vi "模态分析使用版2.vi"() -> ()   [LabVIEW 2014]
uses:
  <vilib>/Analysis/4window.llb/windowTd.ctl
  <vilib>/Utility/error.llb/DialogType.ctl
  <vilib>/DAQmx/read.llb/DAQmx Read (Analog 1D Wfm NChan NSamp).vi
  <vilib>/DAQmx/create/channels.llb/DAQmx Create Channel (AI-Voltage-Basic).vi
  <vilib>/DAQmx/configure/timing.llb/DAQmx Timing (Sample Clock).vi
  <vilib>/DAQmx/miscellaneous.llb/DAQmx Fill In Error Info.vi
  <vilib>/Waveform/WDTOps.llb/WDT Number of Waveform Samples DBL.vi
  <vilib>/Waveform/WDTOps.llb/WDT Append Waveforms DBL.vi
  <vilib>/Waveform/WDTOps.llb/WDT Get Waveform Subset DBL.vi
  <vilib>/Analysis/NI_AALPro.lvlib
panel:
  out "FRF magnifitude":cluster{"f0":dbl, "df":dbl, "magnitude":dbl[]}(graph)
  out "相关函数":cluster{"f0":dbl, "df":dbl, "magnitude":dbl[]}(graph)
  out "FRF Phase":cluster{"f0":dbl, "df":dbl, "magnitude":dbl[]}(graph)
  in  "DAQmx物理通道":tag
  in  "input terminal configuration 2":i32(ring)=-1 caption="输入接线端配置" items=["默认"=-1, "RSE"=10083, "NRSE"=10078, "差分"=10106, "伪差分"=12529]
  in  "DAQmx物理通道 2":tag
  in  "input terminal configuration 3":i32(ring)=-1 caption="输入接线端配置" items=["默认"=-1, "RSE"=10083, "NRSE"=10078, "差分"=10106, "伪差分"=12529]
  in  "rate 2":dbl=1000.0 caption="速率" format="%0.2f"
  in  "sample mode 2":i32(ring)=10178 caption="采样模式" items=["有限采样"=10178, "连续采样"=10123, "硬件定时单点"=12522]
  in  "number of samples per channel 2":i32=-1 caption="每通道采样数"
  in  "最小采集电压值 2":dbl=-10.0 format="%#_g  V"
  in  "最大采集电压值  2":dbl=10.0 format="%#_g  V"
  in  "units 2":i32(ring)=10348 caption="单位" items=["伏特"=10348, "来自自定义换算"=10065]
  in  "units 3":i32(ring)=10348 caption="单位" items=["伏特"=10348, "来自自定义换算"=10065]
  in  "averaging parameters":T1={"averaging mode"=enum."No averaging", "weighting mode"=enum."Exponential", "number of averages"=10} caption="平均参数" {"number of averages" min=1}
  in  "window":T2=1 caption="窗" items=["矩形"=0, "Hanning"=1, "Hamming"=2, "Blackman-Harris"=3, "Exact Blackman"=4, "Blackman"=5, "Flat Top"=6, "4阶Blackman-Harris "=7, "7阶Blackman-Harris"=8, "Low Sidelobe"=9, "Blackman Nuttall"=11, "三角"=30, "Bartlett-Hanning"=31, "Bohman"=32, "Parzen"=33, "Welch"=34, "Kaiser"=60, "Dolph-Chebyshev"=61, "高斯"=62]
  in  "view":T3 caption="查看"
  in  "FRF Mode":enum16{"H1", "H2", "H3"}(ring) caption="FRF模式"
  in  "删除上一次波形":bool
  out "激振信号":waveform(dbl)(graph)
  out "响应信号":waveform(dbl)(graph)
  out "激振信号 3":waveform(dbl)[](graph)
  in  "数值":i32
  out "激振信号 4":waveform(dbl)[](graph)
  in  "阈值":dbl=-1.0
  in  "预触发长度":i32=-1
  in  "激振通道":i32=-1
  in  "激振传感器灵敏度":dbl=-1.0
  in  "采集次数":i32=-1 caption="预触发长度"
  in  "停止按钮":bool
  in  "激振计数":i32=-1 caption="预触发长度"
  out "激振信号 2":waveform(dbl)[](graph)
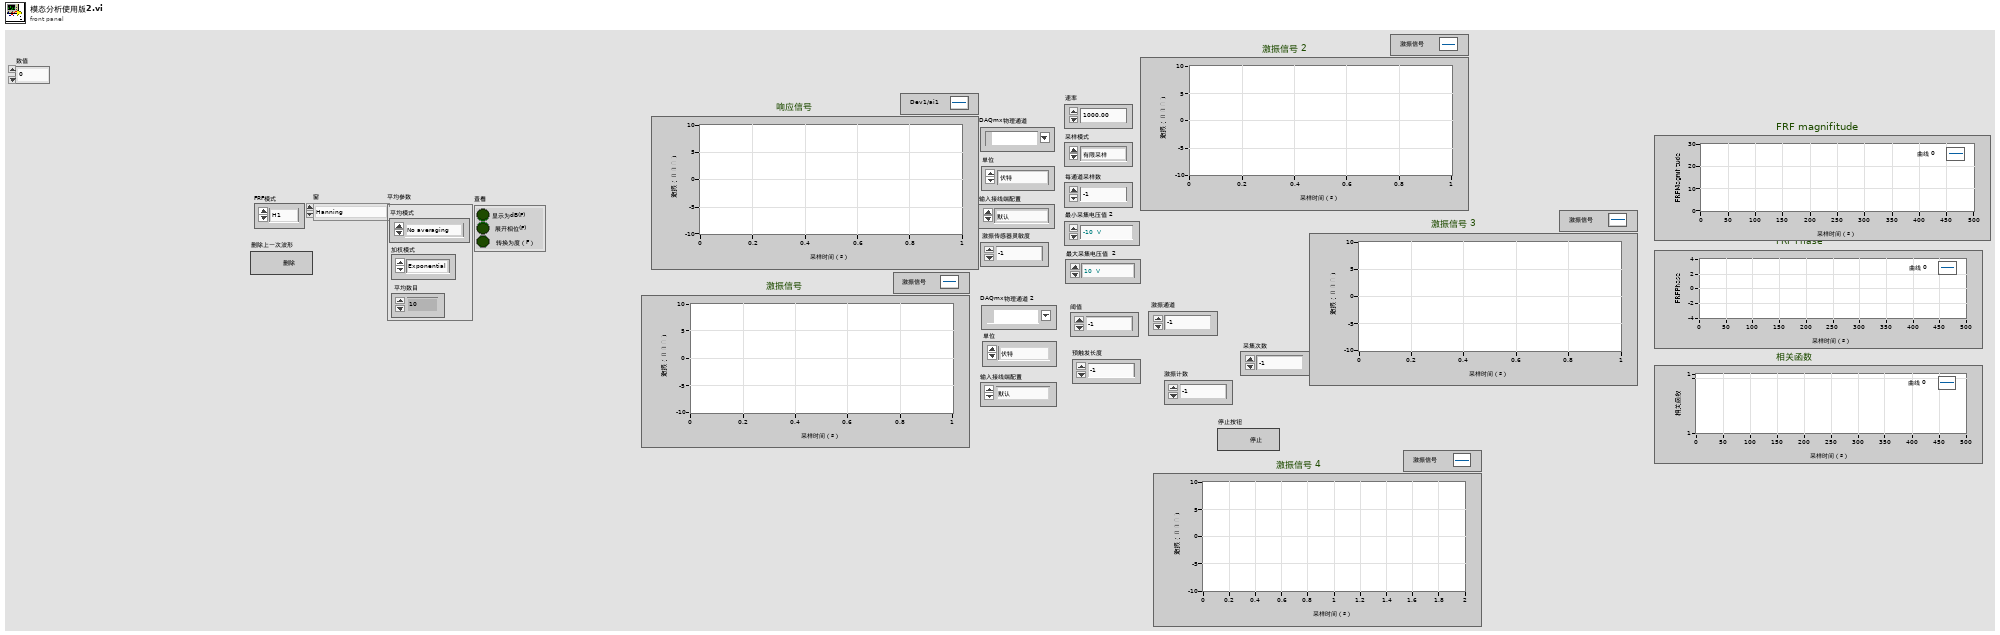
[diagram p1: front panel]
types:
  T1 = cluster{"averaging mode":enum16{"No averaging", "Vector averaging", "RMS averaging", "Peak hold"}, "weighting mode":enum16{"Linear", "Exponential"}, "number of averages":u32}
  T2 = typedef "NI_AALPro.lvlib/windowTd.ctl" = u32
  T3 = cluster{"dB On (F)":bool, "unwrap phase (F)":bool, "convert to degree (F)":bool}
  T4 = typedef "DialogType.ctl" = u16
  T5 = cluster{"magnitude":cluster{"f0":dbl, "df":dbl, "magnitude":dbl[]}, "phase":cluster{"f0":dbl, "df":dbl, "phase":dbl[]}, "coherence":cluster{"f0":dbl, "df":dbl, "coherence":dbl[]}}
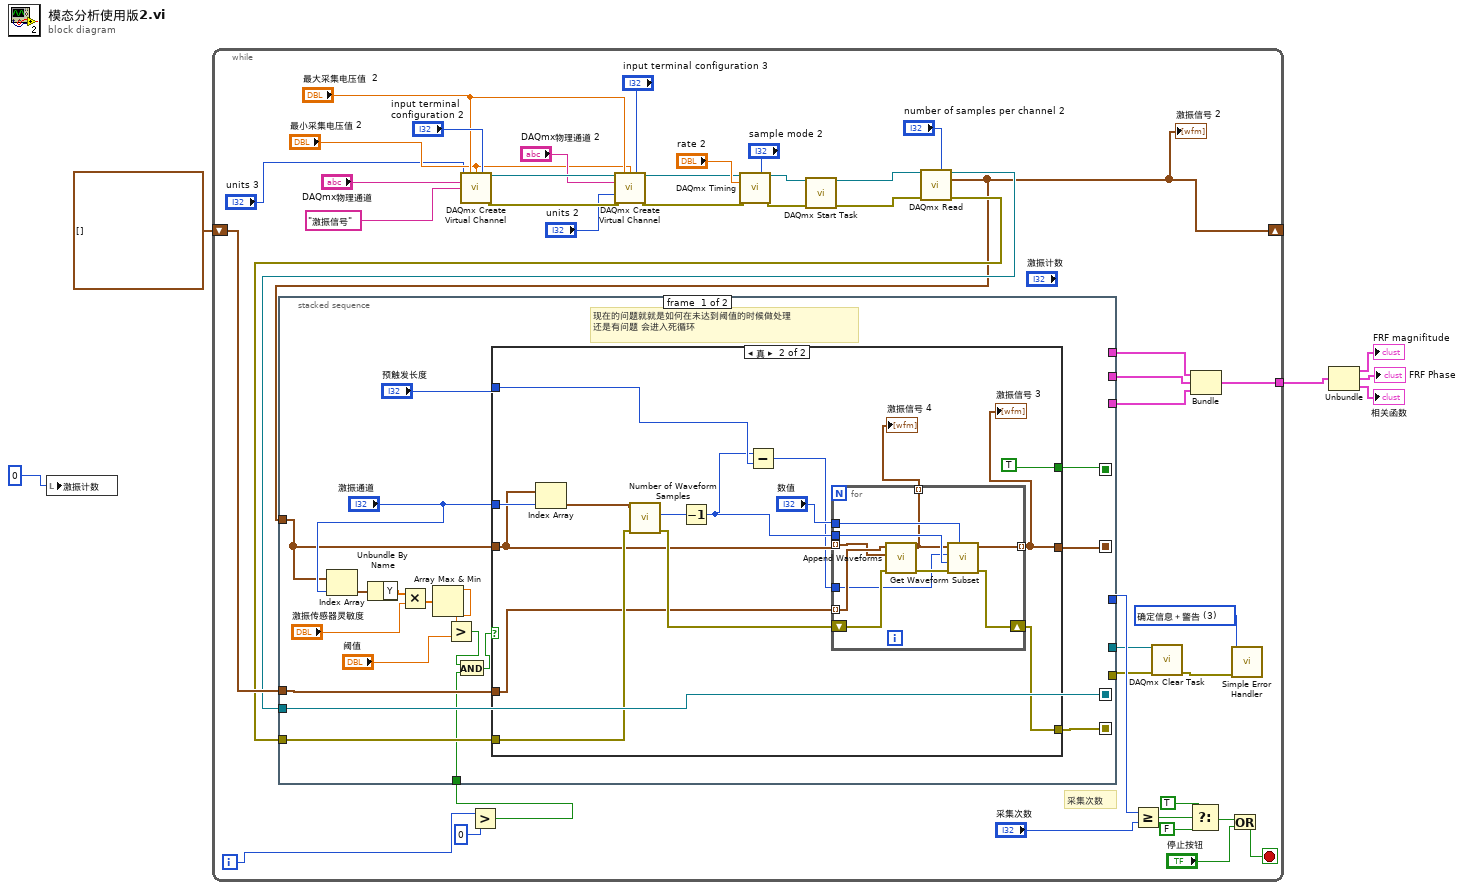
[diagram p0: block diagram]
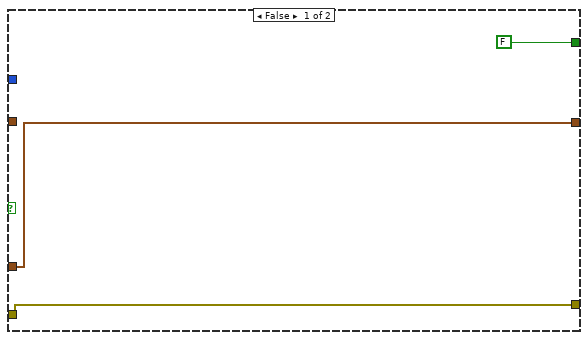
[diagram p2: hidden frame]
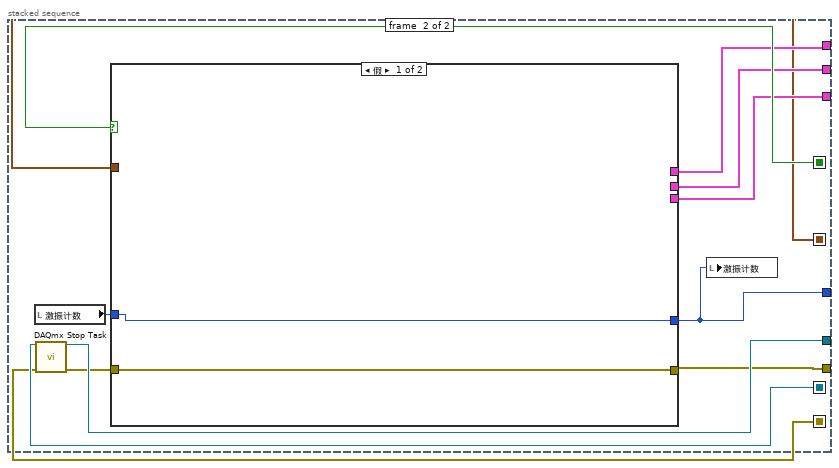
[diagram p3: hidden frame]
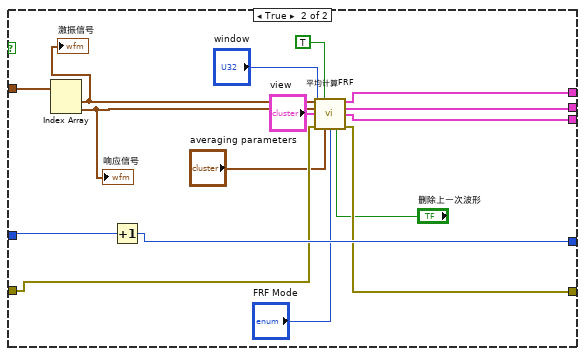
[diagram p4: hidden frame]
diagram:
  n1 = local write "激振计数"(0) -> ()
  n2 = while {
    shift-right: [w10] -> _
    shift-left: waveform(dbl)[] [] ("data") -> [w27]
    tunnel: [w14] -> w1
    i -> [w8]
    stop <- w12 stop-if-true
    w39 = T4 3 items=["无对话框", "确定信息", "继续或停止信息", "确定信息＋警告", "继续/停止+警告"] ("type of dialog (OK msg:1)")
    # "采集次数"
    n3 = call-poly <vilib>:"DAQmx Create Virtual Channel.vi"("maximum value"="最大采集电压值  2", "minimum value"="最小采集电压值 2", "input terminal configuration"="input terminal configuration 2", "physical channels"="DAQmx物理通道", "name to assign"="激振信号", "units"="units 3") -> ("task out"=w46:refnum<k21>, "error out"=w45:errorcluster)  [unwired: 8 in]
    n4 = Greater?(x=w8, y=0) -> (0:w7:bool)
    n5 = call-poly <vilib>:"DAQmx Create Virtual Channel.vi"("task in"=w46, "maximum value"="最大采集电压值  2", "minimum value"="最小采集电压值 2", "input terminal configuration"="input terminal configuration 3", "physical channels"="DAQmx物理通道 2", "units"="units 2", "error in"=w45) -> ("task out"=w36:refnum<k21>, "error out"=w35:errorcluster)  [unwired: 7 in]
    n6 = call-poly <vilib>:"DAQmx Timing.vi"("task/channels in"=w36, "sample mode"="sample mode 2", "rate"="rate 2", "error in"=w35) -> ("task out"=w41:refnum<k21>, "error out"=w40:errorcluster)  [unwired: 10 in]
    n7 = call <vilib>:"DAQmx Start Task.vi"("task/channels in"=w41, "error in"=w40) -> ("task out"=w31:refnum<k21>, "error out"=w30:errorcluster)  [unwired: 12 in]
    n8 = call-poly <vilib>:"DAQmx Read.vi"("task/channels in"=w31, "number of samples per channel"="number of samples per channel 2", "error in"=w30) -> ("task out"=w25:refnum<k21>, "data"=w10:waveform(dbl)[], "error out"=w26:errorcluster)  [unwired: 10 in]
    "激振信号 2" <- w10
    n9 = stacked-sequence {
      seq-local: [w59 _] -> [_ w107]
      seq-local: [w58 _] -> [_ w96]
      seq-local: [w57 _] -> [_ w105]
      seq-local: [w55 _] -> [_ w106]
      tunnel: w10 -> [w54 _]
      tunnel: w27 -> [w67 _]
      tunnel: w26 -> [w56 _]
      tunnel: w25 -> [w55 _]
      tunnel: [_ w104] -> w20
      tunnel: [_ w97] -> w21
      tunnel: [_ w101] -> w18
      tunnel: [_ w100] -> w17
      tunnel: [_ w99] -> w16
      tunnel: [_ w98] -> w15
      tunnel: w7 -> [w52 _]
      frame #0 {
        # "现在的问题就就是如何在未达到阈值的时候做处理\n还是有问题 会进入死循环"
        n10 = Index Array(array=w54, index="激振通道") -> (element=w65:waveform(dbl))
        n11 = Unbundle By Name(w65) -> ("Y"=w64:dbl[])
        n12 = Multiply(x=w64, y="激振传感器灵敏度") -> (x*y=w61:dbl[])
        n13 = Array Max & Min(array=w61) -> (max value=w60:dbl)  [unwired: 3 out]
        n14 = Greater?(x=w60, y="阈值") -> (0:w51:bool)
        n15 = And(x=w51, y=w52) -> (x .and. y?=w50:bool)
        n16 = case shown="真" w50 {
          tunnel: w54 -> [_ w76]
          tunnel: "激振通道" -> [_ w85]
          tunnel: w56 -> [w70 w83]
          tunnel: "预触发长度" -> [_ w74]
          tunnel: w67 -> [w68 w75]
          tunnel: [w70 w81] -> w57
          tunnel: [w68 w79] -> w58
          tunnel: [FALSE TRUE] -> w59
          frame False {
          }
          frame True {
            n17 = Index Array(array=w76, index=w85) -> (element=w78:waveform(dbl))
            n18 = call-poly <vilib>:"Number of Waveform Samples.vi"("error in (no error)"=w83, "waveform in"=w78) -> ("error out"=w82:errorcluster, "number of samples"=w84:i32)  [unwired: 7 in, 1 out]
            n19 = Decrement(x=w84) -> (x-1=w73:i32)
            n20 = Subtract(x=w73, y=w74) -> (x-y=w72:i32)
            n21 = for {
              shift-right: [w90] -> w81
              shift-left: w82 -> [w93]
              tunnel: w76 -> [w94] mode=indexing
              tunnel: [w91] -> w79 mode=indexing
              tunnel: "数值" -> [w88]
              tunnel: w75 -> [w95] mode=indexing
              tunnel: w72 -> [w86]
              tunnel: w73 -> [w89]
              tunnel: [w87] -> w71 mode=indexing
              n22 = call-poly <vilib>:"Append Waveforms.vi"("error in (no error)"=w93, "waveform B"=w94, "waveform A"=w95) -> ("error out"=w92:errorcluster, "waveform out"=w87:waveform(dbl))  [unwired: 7 in]
              n23 = call-poly <vilib>:"Get Waveform Subset.vi"("start/duration format"=w88, "error in (no error)"=w92, "duration"=w89, "start samples/time"=w86, "waveform in"=w87) -> ("error out"=w90:errorcluster, "waveform out"=w91:waveform(dbl))  [unwired: 1 in, 2 out]
            }
            "激振信号 3" <- w79
            "激振信号 4" <- w71
          }
        }
      }
      frame #1 {
        n24 = local read "激振计数"() -> (w102:i32)
        n25 = call <vilib>:"DAQmx Stop Task.vi"("task/channels in"=w106, "error in"=w105) -> ("task out"=w104:refnum<k21>, "error out"=w103:errorcluster)  [unwired: 12 in]
        n26 = case shown="假" w107 {
          tunnel: w96 -> [_ w112]
          tunnel: w103 -> [w108 w123]
          tunnel: w102 -> [w109 w125]
          tunnel: [w109 w124] -> w97
          tunnel: [w108 w122] -> w101
          tunnel: [_ w115] -> w100
          tunnel: [_ w114] -> w99
          tunnel: [_ w113] -> w98
          frame False {
          }
          frame True {
            n27 = Index Array(array=w112) -> (element #1=w111:waveform(dbl), element #2=w110:waveform(dbl))  [unwired: 2 in]
            "激振信号" <- w111
            "响应信号" <- w110
            n28 = Increment(x=w125) -> (x+1=w124:i32)
            n29 = call "平均计算FRF.vi"("time signal X"=w111, "restart averaging (F)"=TRUE, "time signal Y"=w110, "window"="window", "view"="view", "error in (no error)"=w123, "averaging parameters"="averaging parameters", "FRF Mode"="FRF Mode", "删除上一波形"="删除上一次波形") -> ("magnitude"=w115:cluster{"f0":dbl, "df":dbl, "magnitude":dbl[]}, "phase"=w114:cluster{"f0":dbl, "df":dbl, "phase":dbl[]}, "coherence"=w113:cluster{"f0":dbl, "df":dbl, "coherence":dbl[]}, "error out"=w122:errorcluster)  [unwired: 1 in, 2 out]
          }
        }
        n30 = local write "激振计数"(w97) -> ()
      }
    }
    n31 = Greater Or Equal?(x=w21, y="采集次数") -> (x >= y?=w24:bool)
    n32 = call <vilib>:"DAQmx Clear Task.vi"("task in"=w20, "error in"=w18) -> ("error out"=w38:errorcluster)  [unwired: 13 in]
    n33 = Select(t=TRUE, s=w24, f=FALSE) -> (s? t:f=w13:bool)
    n34 = Bundle("magnitude"=w17, "phase"=w16, "coherence"=w15) -> (w14:T5)  [unwired: 1 in]
    n35 = Or(x=w13, y="停止按钮") -> (x .or. y?=w12:bool)
    n36 = call <vilib>:"Simple Error Handler.vi"("type of dialog (OK msg:1)"=w39, "error in (no error)"=w38) -> ()  [unwired: 3 in, 5 out]
  }
  n37 = Unbundle(w1) -> ("magnitude"=→"FRF magnifitude":cluster{"f0":dbl, "df":dbl, "magnitude":dbl[]}, "phase"=→"FRF Phase":cluster{"f0":dbl, "df":dbl, "phase":dbl[]}, "coherence"=→"相关函数":cluster{"f0":dbl, "df":dbl, "coherence":dbl[]})
